vi "SignalSenderLoop.TestLauncher.vi"() -> ()   [LabVIEW 2020, in "SignalSenderLoop.lvclass"]
doc: "JKI State Machine Objects (SMO) 1.0.0.5\nJKI - JKI\nCopyright (c) 2016, JKI"
uses:
  SignalSenderLoop.lvclass
  Typedefs/Data.ctl
  C:/Program Files (x86)/National Instruments/LabVIEW 2020/vi.lib/JKI/JKI SMO/SMO/SMO.lvclass
  Typedefs/PublicEvents--Cluster.ctl
  Typedefs/SetpointChanged--EventData--Cluster.ctl
  <vilib>/JKI/JKI SMO/SMO/Typedefs/Public Events.ctl
  <vilib>/JKI/JKI SMO/SMO/Typedefs/SMOState --Enum.ctl
  <vilib>/JKI/JKI SMO/SMO/Typedefs/Reserve State--Enum.ctl
  <vilib>/JKI/JKI SMO/SMO/SMO.lvclass
panel:
  out "SMOArry":refnum<class "SignalSenderLoop.lvclass">[](array[class])
  out "EventHandl(订阅事件用)":refnum<event-registration>[](array[refnum])
  in  "SignalsSet 2":dbl[](array[numeric])=[0.0]
  out "元素":refnum<class "SignalSenderLoop.lvclass">
  in  "SignalsSet":dbl[](array[numeric])=[60.0, 1.0]
  out "Value 3":T1
  out "Value 2":T1
  out "数组":errorcluster[](array[cluster])
  out "Value":T1
  in  "Setpoint":dbl(slide) scale=0.0..10.0
  out "error out":errorcluster
  in  "Stop":bool
  # "ECU Signals Sender Test Launcher"
  # "数组为空，不发送任何帧，即停止发送"
  # "数组为空，不发送任何帧，即停止发送"
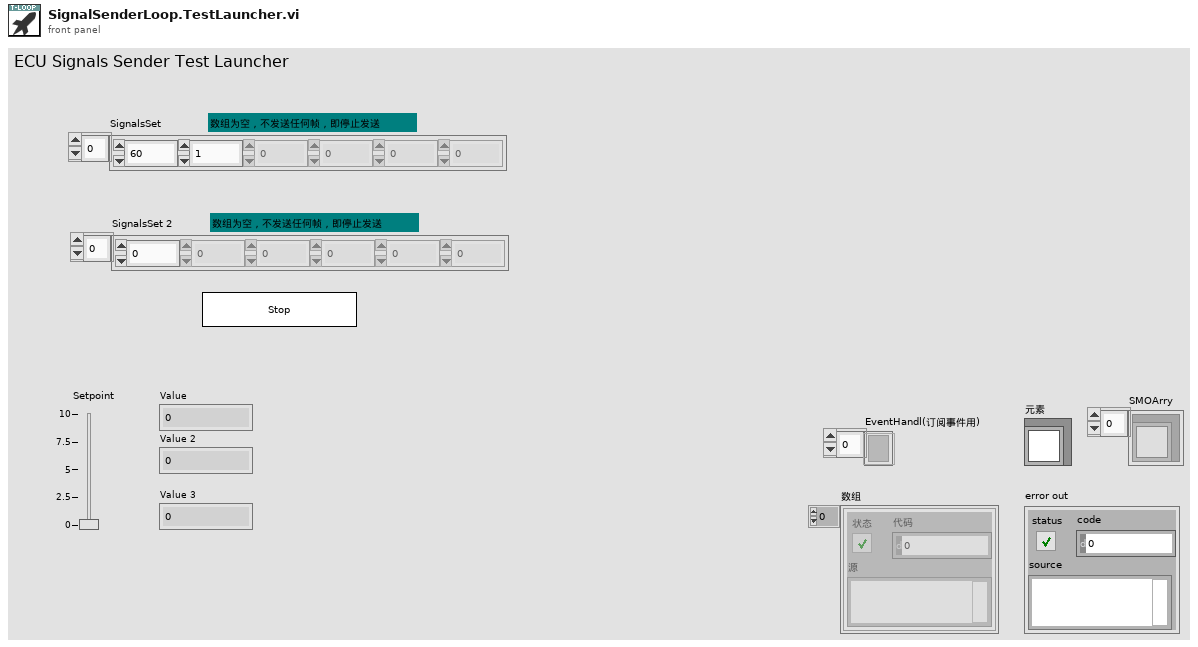
[diagram p1: front panel]
types:
  T1 = typedef "SignalSenderLoop.lvclass/Data.ctl" = dbl
  T2 = typedef "SMO.lvclass/SMOState --Enum.ctl" = enum16{"unknown", "Created", "Started", "Stopped"}
  T3 = typedef "SMO.lvclass/Public Events.ctl" = cluster{"Error":refnum<user-event>, "State":refnum<user-event>, "Reserve State":refnum<user-event>}
  T4 = typedef "SignalSenderLoop.lvclass/PublicEvents--Cluster.ctl" = cluster{"Setpoint Changed":refnum<user-event>, "Value Changed":refnum<user-event>}
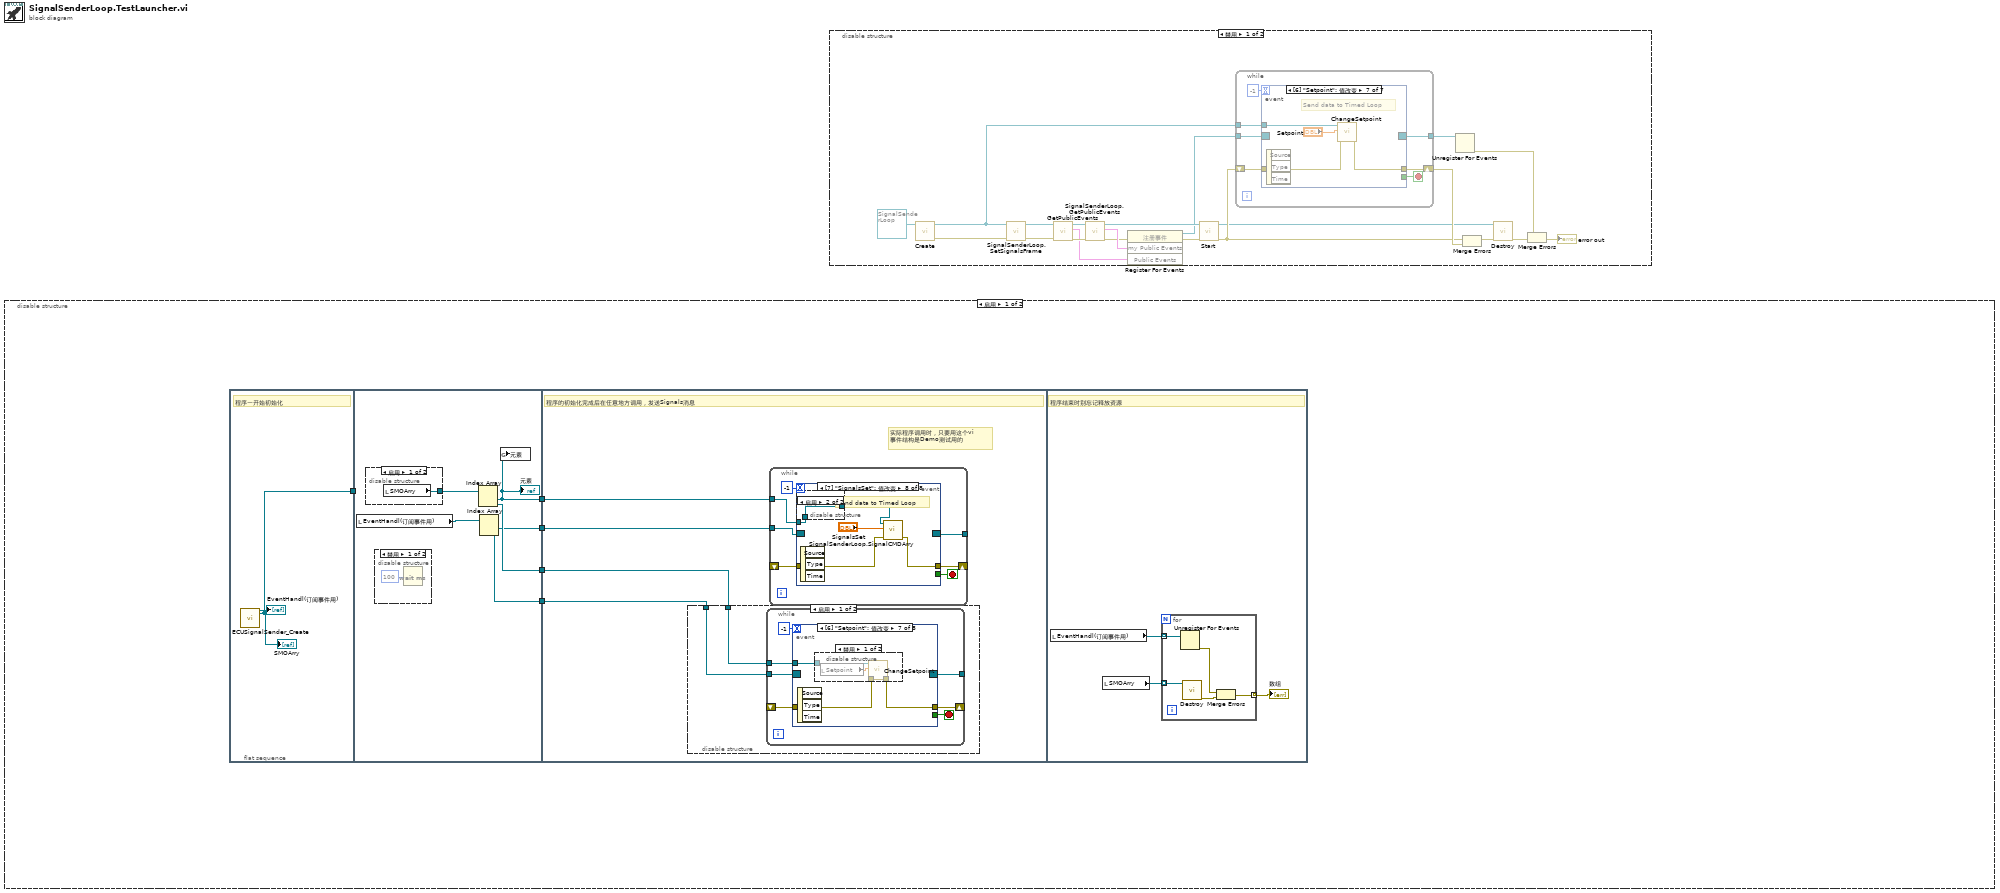
[diagram p0: block diagram]
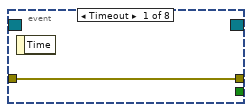
[diagram p4: hidden frame]
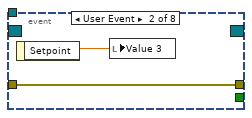
[diagram p5: hidden frame]
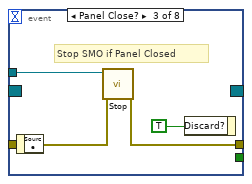
[diagram p6: hidden frame]
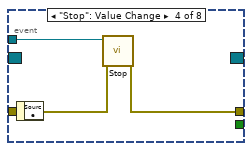
[diagram p7: hidden frame]
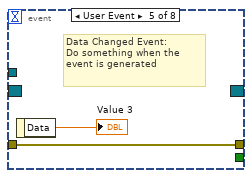
[diagram p8: hidden frame]
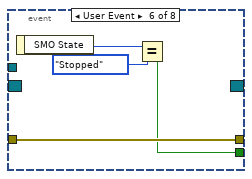
[diagram p9: hidden frame]
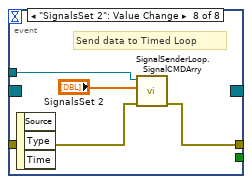
[diagram p11: hidden frame]
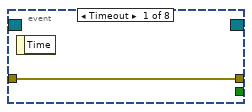
[diagram p13: hidden frame]
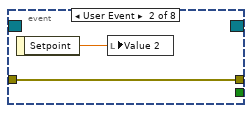
[diagram p14: hidden frame]
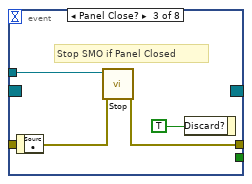
[diagram p15: hidden frame]
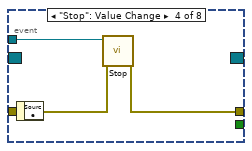
[diagram p16: hidden frame]
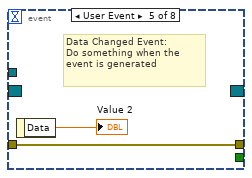
[diagram p17: hidden frame]
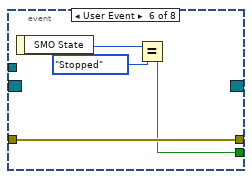
[diagram p18: hidden frame]
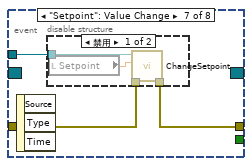
[diagram p19: hidden frame]
diagram:
  n1 = disable-structure shown="启用" {
    frame Enabled {
      n2 = flat-sequence {
        tunnel: [w6] -> w1
        tunnel: [w8] -> w5
        tunnel: [w11] -> w4
        tunnel: [w10] -> w3
        tunnel: [w9] -> w2
        tunnel: w1 -> [_]
        tunnel: w5 -> [w20]
        tunnel: w4 -> [w19]
        tunnel: w3 -> [w18]
        tunnel: w2 -> [w17]
        frame #0 {
          # "程序一开始初始化"
          n3 = call "ECUSignalSender_Create.vi"() -> ("EventHandl(订阅事件用)"=→"EventHandl(订阅事件用)":refnum<event-registration>[], "SMOArry"=w6:refnum<class "SignalSenderLoop.lvclass">[])  [unwired: 17 in, 1 out]
          "SMOArry" <- w6
        }
        frame #1 {
          n4 = local read "EventHandl(订阅事件用)"() -> (w12:refnum<event-registration>[])
          n5 = disable-structure shown="启用" {
            disable-tunnel: [w14 w15] -> w13
            frame Enabled {
              n6 = local read "SMOArry"() -> (w14:refnum<class "SignalSenderLoop.lvclass">[])
            }
            frame Disabled {
            }
          }
          n7 = disable-structure shown="禁用" {
            frame Disabled {
              n8 = Wait (ms)(milliseconds to wait=u32 100 ("等待时间（毫秒）")) -> ()  [unwired: 1 out]
            }
            frame Enabled {
            }
          }
          n9 = Index Array(array=w13) -> (element #1=w8:refnum<class "SignalSenderLoop.lvclass">, element #2=w11:refnum<class "SignalSenderLoop.lvclass">)  [unwired: 2 in]
          "元素" <- w8
          n10 = Index Array(array=w12) -> (element #1=w10:refnum<event-registration>, element #2=w9:refnum<event-registration>)  [unwired: 2 in]
          n11 = global write "test 1.vi" "元素"(w8) -> ()
        }
        frame #2 {
          # "实际程序调用时，只要用这个vi\n事件结构是Demo测试用的"
          # "程序的初始化完成后在任意地方调用，发送Signals消息"
          n12 = disable-structure shown="启用" {
            disable-tunnel: w17 -> [w22 _]
            disable-tunnel: w19 -> [w21 _]
            frame Enabled {
              n13 = while {
                shift-right: [w28] -> _
                shift-left: _ -> [w27]
                tunnel: w22 -> [w26]
                tunnel: [w25] -> _
                tunnel: w21 -> [w24]
                stop <- w29 stop-if-true
                n14 = event shown="[6] \"Setpoint\": 值改变" {
                  selector: w26 -> [_ _ _ _ _ _ _ _]
                  dyn-events: [_ _ _ _ _ _ _ _] -> w25
                  timeout: -1 -> [_ _ _ _ _ _ _ _]
                  tunnel: [_ _ _ _ _ w42 _ _] -> w29
                  tunnel: w24 -> [_ _ w36 w39 _ _ w48 w56]
                  tunnel: [w30 w32 w35 w38 w41 w45 w46 w53] -> w28
                  tunnel: w27 -> [w30 w32 w34 w37 w41 w45 w47 w54]
                  event Timeout {
                    n15 = event-data() -> ()  [unwired: 1 in, 1 out]
                  }
                  event User Event {
                    n16 = event-data() -> ("Setpoint"=w31:T1)  [unwired: 1 in]
                    n17 = local write "Value 3"(w31) -> ()
                  }
                  event Panel Close? {
                    # "Stop SMO if Panel Closed"
                    n18 = event-data() -> ()  [unwired: 1 in, 1 out]
                    n19 = call <vilib>:"Stop.vi"("error in (no error)"=w34, "SMO"=w36) -> ("error out"=w35:errorcluster)  [unwired: 8 in, 1 out]
                    n20 = event-data("Discard?"=TRUE ("OK")) -> ()  [unwired: 1 in, 1 out]
                  }
                  event "Stop": Value Change {
                    n21 = event-data() -> ()  [unwired: 1 in, 1 out]
                    n22 = call <vilib>:"Stop.vi"("error in (no error)"=w37, "SMO"=w39) -> ("error out"=w38:errorcluster)  [unwired: 8 in, 1 out]
                  }
                  event User Event {
                    # "Data Changed Event:\nDo something when the\nevent is generated"
                    n23 = event-data() -> ("Data"=→"Value 3":T1)  [unwired: 1 in]
                  }
                  event User Event {
                    n24 = event-data() -> ("SMO State"=w44:T2)  [unwired: 1 in]
                    n25 = Equal?(x=w44, y=SMOState_--Enum."Stopped") -> (x = y?=w42:bool)
                  }
                  event "Setpoint": Value Change {
                    n26 = event-data() -> ()  [unwired: 1 in, 3 out]
                    n27 = disable-structure shown="禁用" {
                      disable-tunnel: w48 -> [w52 _]
                      disable-tunnel: w47 -> [w51 _]
                      disable-tunnel: [w50 _] -> w46
                      frame Disabled {
                        n28 = local read "Setpoint"() -> (w49:dbl)
                        n29 = call "ChangeSetpoint.vi"("error in (no error)"=w51, "Setpoint"=w49, "SignalSenderLoop"=w52) -> ("error out"=w50:errorcluster)  [unwired: 7 in, 1 out]
                      }
                      frame Enabled {
                      }
                    }
                  }
                  event "SignalsSet 2": Value Change {
                    # "Send data to Timed Loop"
                    n30 = event-data() -> ()  [unwired: 1 in, 3 out]
                    n31 = call "SignalSenderLoop.SignalCMDArry.vi"("error in (no error)"=w54, "SignalCMDArry"="SignalsSet 2", "SignalSenderLoop"=w56) -> ("error out"=w53:errorcluster)  [unwired: 7 in, 1 out]
                  }
                }
              }
            }
            frame Disabled {
            }
          }
          n32 = while {
            shift-right: [w62] -> _
            shift-left: _ -> [w61]
            tunnel: [w60] -> _
            tunnel: w20 -> [w58]
            tunnel: w18 -> [w57]
            stop <- w63 stop-if-true
            n33 = event shown="[7] \"SignalsSet\": 值改变" {
              selector: w57 -> [_ _ _ _ _ _ _ _]
              dyn-events: [_ _ _ _ _ _ _ _] -> w60
              timeout: -1 -> [_ _ _ _ _ _ _ _]
              tunnel: [_ _ _ _ _ w76 _ _] -> w63
              tunnel: [w64 w66 w70 w73 w75 w79 w81 w90] -> w62
              tunnel: w61 -> [w64 w66 w69 w72 w75 w79 w82 w91]
              tunnel: w58 -> [_ _ w67 w71 _ _ w80 w87]
              event Timeout {
                n34 = event-data() -> ()  [unwired: 1 in, 1 out]
              }
              event User Event {
                n35 = event-data() -> ("Setpoint"=w65:T1)  [unwired: 1 in]
                n36 = local write "Value 2"(w65) -> ()
              }
              event Panel Close? {
                # "Stop SMO if Panel Closed"
                n37 = event-data() -> ()  [unwired: 1 in, 1 out]
                n38 = call <vilib>:"Stop.vi"("error in (no error)"=w69, "SMO"=w67) -> ("error out"=w70:errorcluster)  [unwired: 8 in, 1 out]
                n39 = event-data("Discard?"=TRUE ("OK")) -> ()  [unwired: 1 in, 1 out]
              }
              event "Stop": Value Change {
                n40 = event-data() -> ()  [unwired: 1 in, 1 out]
                n41 = call <vilib>:"Stop.vi"("error in (no error)"=w72, "SMO"=w71) -> ("error out"=w73:errorcluster)  [unwired: 8 in, 1 out]
              }
              event User Event {
                # "Data Changed Event:\nDo something when the\nevent is generated"
                n42 = event-data() -> ("Data"=→"Value 2":T1)  [unwired: 1 in]
              }
              event User Event {
                n43 = event-data() -> ("SMO State"=w78:T2)  [unwired: 1 in]
                n44 = Equal?(x=w78, y=SMOState_--Enum."Stopped") -> (x = y?=w76:bool)
              }
              event "Setpoint": Value Change {
                n45 = event-data() -> ()  [unwired: 1 in, 3 out]
                n46 = disable-structure shown="禁用" {
                  disable-tunnel: w82 -> [w86 _]
                  disable-tunnel: [w85 _] -> w81
                  disable-tunnel: w80 -> [w83 _]
                  frame Disabled {
                    n47 = local read "Setpoint"() -> (w84:dbl)
                    n48 = call "ChangeSetpoint.vi"("error in (no error)"=w86, "Setpoint"=w84, "SignalSenderLoop"=w83) -> ("error out"=w85:errorcluster)  [unwired: 7 in, 1 out]
                  }
                  frame Enabled {
                  }
                }
              }
              event "SignalsSet": Value Change {
                # "Send data to Timed Loop"
                n49 = disable-structure shown="启用" {
                  disable-tunnel: [w92 w93] -> w88
                  disable-tunnel: w87 -> [_ w93]
                  frame Disabled {
                    n50 = local read "元素"() -> (w92:refnum<class "SignalSenderLoop.lvclass">)
                  }
                  frame Enabled {
                  }
                }
                n51 = event-data() -> ()  [unwired: 1 in, 3 out]
                n52 = call "SignalSenderLoop.SignalCMDArry.vi"("error in (no error)"=w91, "SignalCMDArry"="SignalsSet", "SignalSenderLoop"=w88) -> ("error out"=w90:errorcluster)  [unwired: 7 in, 1 out]
              }
            }
          }
        }
        frame #3 {
          # "程序结束时别忘记释放资源"
          n53 = local read "EventHandl(订阅事件用)"() -> (w95:refnum<event-registration>[])
          n54 = local read "SMOArry"() -> (w94:refnum<class "SignalSenderLoop.lvclass">[])
          n55 = for {
            tunnel: w95 -> [w101] mode=indexing
            tunnel: [w98] -> w96 mode=indexing
            tunnel: w94 -> [w97] mode=indexing
            n56 = Unregister For Events(event registration refnum=w101) -> (error out=w100:errorcluster)  [unwired: 1 in]
            n57 = call <vilib>:"Destroy.vi"("SMO"=w97) -> ("error out"=w99:errorcluster)  [unwired: 10 in]
            n58 = Merge Errors(w100, w99) -> (w98:errorcluster)
          }
          "数组" <- w96
        }
      }
    }
    frame Disabled {
    }
  }
  n59 = disable-structure shown="禁用" {
    frame Disabled {
      n60 = call <vilib>:"Create.vi"("SMO"=refnum<class "SignalSenderLoop.lvclass"> refnum ("SMO.Template.lvclass")) -> ("error out"=w103:errorcluster, "SMO out"=w105:refnum<class "SignalSenderLoop.lvclass">)  [unwired: 8 in, 1 out]
      n61 = call "SignalSenderLoop.SetSignalsFrame.vi"("error in (no error)"=w103, "SignalSenderLoop"=w105) -> ("error out"=w102:errorcluster, "SignalSenderLoop out"=w104:refnum<class "SignalSenderLoop.lvclass">)  [unwired: 8 in]
      n62 = call <vilib>:"GetPublicEvents.vi"("error in (no error)"=w102, "SMO"=w104) -> ("error out"=w111:errorcluster, "Public Events"=w107:T3, "SMO out"=w110:refnum<class "SignalSenderLoop.lvclass">)  [unwired: 7 in]
      n63 = call "SignalSenderLoop.GetPublicEvents.vi"("error in (no error)"=w111, "SignalSenderLoop"=w110) -> ("error out"=w109:errorcluster, "my Public Events"=w112:T4, "SignalSenderLoop out"=w113:refnum<class "SignalSenderLoop.lvclass">)  [unwired: 7 in]
      n64 = register-events(error in=w109, w112, w107) -> (reference out=w106:refnum<event-registration>, error out=w108:errorcluster)  [unwired: 1 in]
      n65 = call <vilib>:"Start.vi"("error in (no error)"=w108, "SMO"=w113) -> ("error out"=w116:errorcluster, "SMO out"=w114:refnum<class "SignalSenderLoop.lvclass">)  [unwired: 8 in]
      n66 = while {
        shift-right: [w128] -> w121
        shift-left: w116 -> [w127]
        tunnel: w106 -> [w126]
        tunnel: [w125] -> w122
        tunnel: w105 -> [w124]
        stop <- w129 stop-if-true
        n67 = event shown="[6] \"Setpoint\": 值改变" {
          selector: w126 -> [_ _ _ _ _ _ _]
          dyn-events: [_ _ _ _ _ _ _] -> w125
          timeout: -1 -> [_ _ _ _ _ _ _]
          tunnel: [_ _ _ _ _ w142 _] -> w129
          tunnel: w124 -> [_ _ w136 w139 _ _ w149]
          tunnel: [w130 w132 w135 w138 w141 w145 w146] -> w128
          tunnel: w127 -> [w130 w132 w134 w137 w141 w145 w147]
          event Timeout {
            n68 = event-data() -> ()  [unwired: 1 in, 1 out]
          }
          event User Event {
            n69 = event-data() -> ("Setpoint"=w131:T1)  [unwired: 1 in]
            n70 = local write "Setpoint"(w131) -> ()
          }
          event Panel Close? {
            # "Stop SMO if Panel Closed"
            n71 = event-data() -> ()  [unwired: 1 in, 1 out]
            n72 = call <vilib>:"Stop.vi"("error in (no error)"=w134, "SMO"=w136) -> ("error out"=w135:errorcluster)  [unwired: 8 in, 1 out]
            n73 = event-data("Discard?"=TRUE ("OK")) -> ()  [unwired: 1 in, 1 out]
          }
          event "Stop": Value Change {
            n74 = event-data() -> ()  [unwired: 1 in, 1 out]
            n75 = call <vilib>:"Stop.vi"("error in (no error)"=w137, "SMO"=w139) -> ("error out"=w138:errorcluster)  [unwired: 8 in, 1 out]
          }
          event User Event {
            # "Data Changed Event:\nDo something when the\nevent is generated"
            n76 = event-data() -> ("Data"=→"Value":T1)  [unwired: 1 in]
          }
          event User Event {
            n77 = event-data() -> ("SMO State"=w144:T2)  [unwired: 1 in]
            n78 = Equal?(x=w144, y=SMOState_--Enum."Stopped") -> (x = y?=w142:bool)
          }
          event "Setpoint": Value Change {
            # "Send data to Timed Loop"
            n79 = event-data() -> ()  [unwired: 1 in, 3 out]
            n80 = call "ChangeSetpoint.vi"("error in (no error)"=w147, "Setpoint"="Setpoint", "SignalSenderLoop"=w149) -> ("error out"=w146:errorcluster)  [unwired: 7 in, 1 out]
          }
        }
      }
      n81 = Unregister For Events(event registration refnum=w122) -> (error out=w120:errorcluster)  [unwired: 1 in]
      n82 = Merge Errors(w116, w121) -> (w115:errorcluster)
      n83 = call <vilib>:"Destroy.vi"("error in (no error)"=w115, "SMO"=w114) -> ("error out"=w118:errorcluster)  [unwired: 9 in]
      n84 = Merge Errors(w120, w118) -> (→"error out":errorcluster)
    }
    frame Enabled {
    }
  }
